vi "Gasringverdichter Test.vi"(6 "Aktion":enum16{"lesen", "Manuell B", "Speed", "init"}(ring), 9 "Speed":u16, 11 "Manueller Betrieb":bool) -> (1 "Speed":u16, 3 "Manueller Betrieb":bool)   [LabVIEW 2020, in "Erweiterte Konfig.lvlib"]
uses:
  Erweiterte Konfig.lvlib
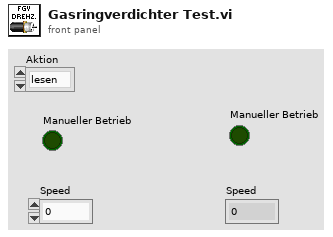
[diagram p1: front panel]
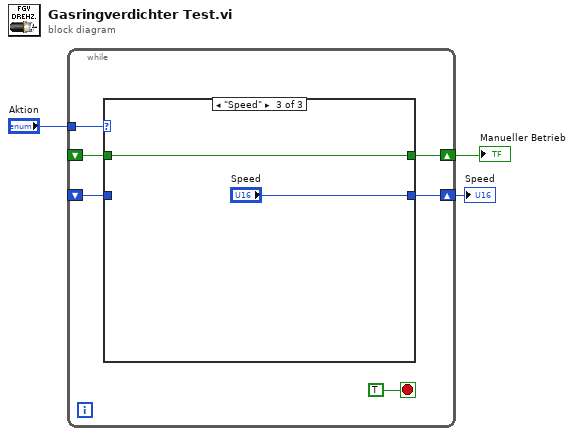
[diagram p0: block diagram]
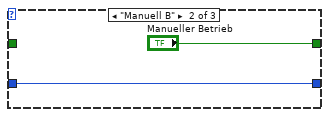
[diagram p3: hidden frame]
diagram:
  n1 = while {
    tunnel: "Aktion" -> [w8]
    shift-right: [w7] -> w2
    shift-left: _ -> [w6]
    shift-right: [w5] -> w1
    shift-left: _ -> [w4]
    stop <- TRUE stop-if-true
    n2 = case shown="\"Speed\"" w8 {
      tunnel: [w11 "Manueller Betrieb" w15] -> w7
      tunnel: w6 -> [w11 _ w15]
      tunnel: [w10 w12 "Speed"] -> w5
      tunnel: w4 -> [w10 w12 _]
      frame "lesen", Default {
      }
      frame "Manuell B" {
      }
      frame "Speed" {
      }
    }
  }
  "Manueller Betrieb" <- w2
  "Speed" <- w1
